vi "CleanDefaultInterfaces.vi"(8 "error in":errorcluster, 11 "Config in":T1) -> (0 "error out":errorcluster, 3 "Config out":T1)   [LabVIEW 2020]
uses:
  <vilib>/WebServerConfig/Config.ctl
  <vilib>/WebServerConfig/Server.ctl
  <vilib>/WebServerConfig/Alias.ctl
  <vilib>/WebServerConfig/ErrorDocument.ctl
  <vilib>/WebServerConfig/Action.ctl
  <vilib>/WebServerConfig/Redirect.ctl
  <vilib>/WebServerConfig/Interface.ctl
  <vilib>/WebServerConfig/AddHandler.ctl
  <vilib>/WebServerConfig/SSL.ctl
  <vilib>/WebServerConfig/CustomLog.ctl
  <vilib>/WebServerConfig/LoadModule.ctl
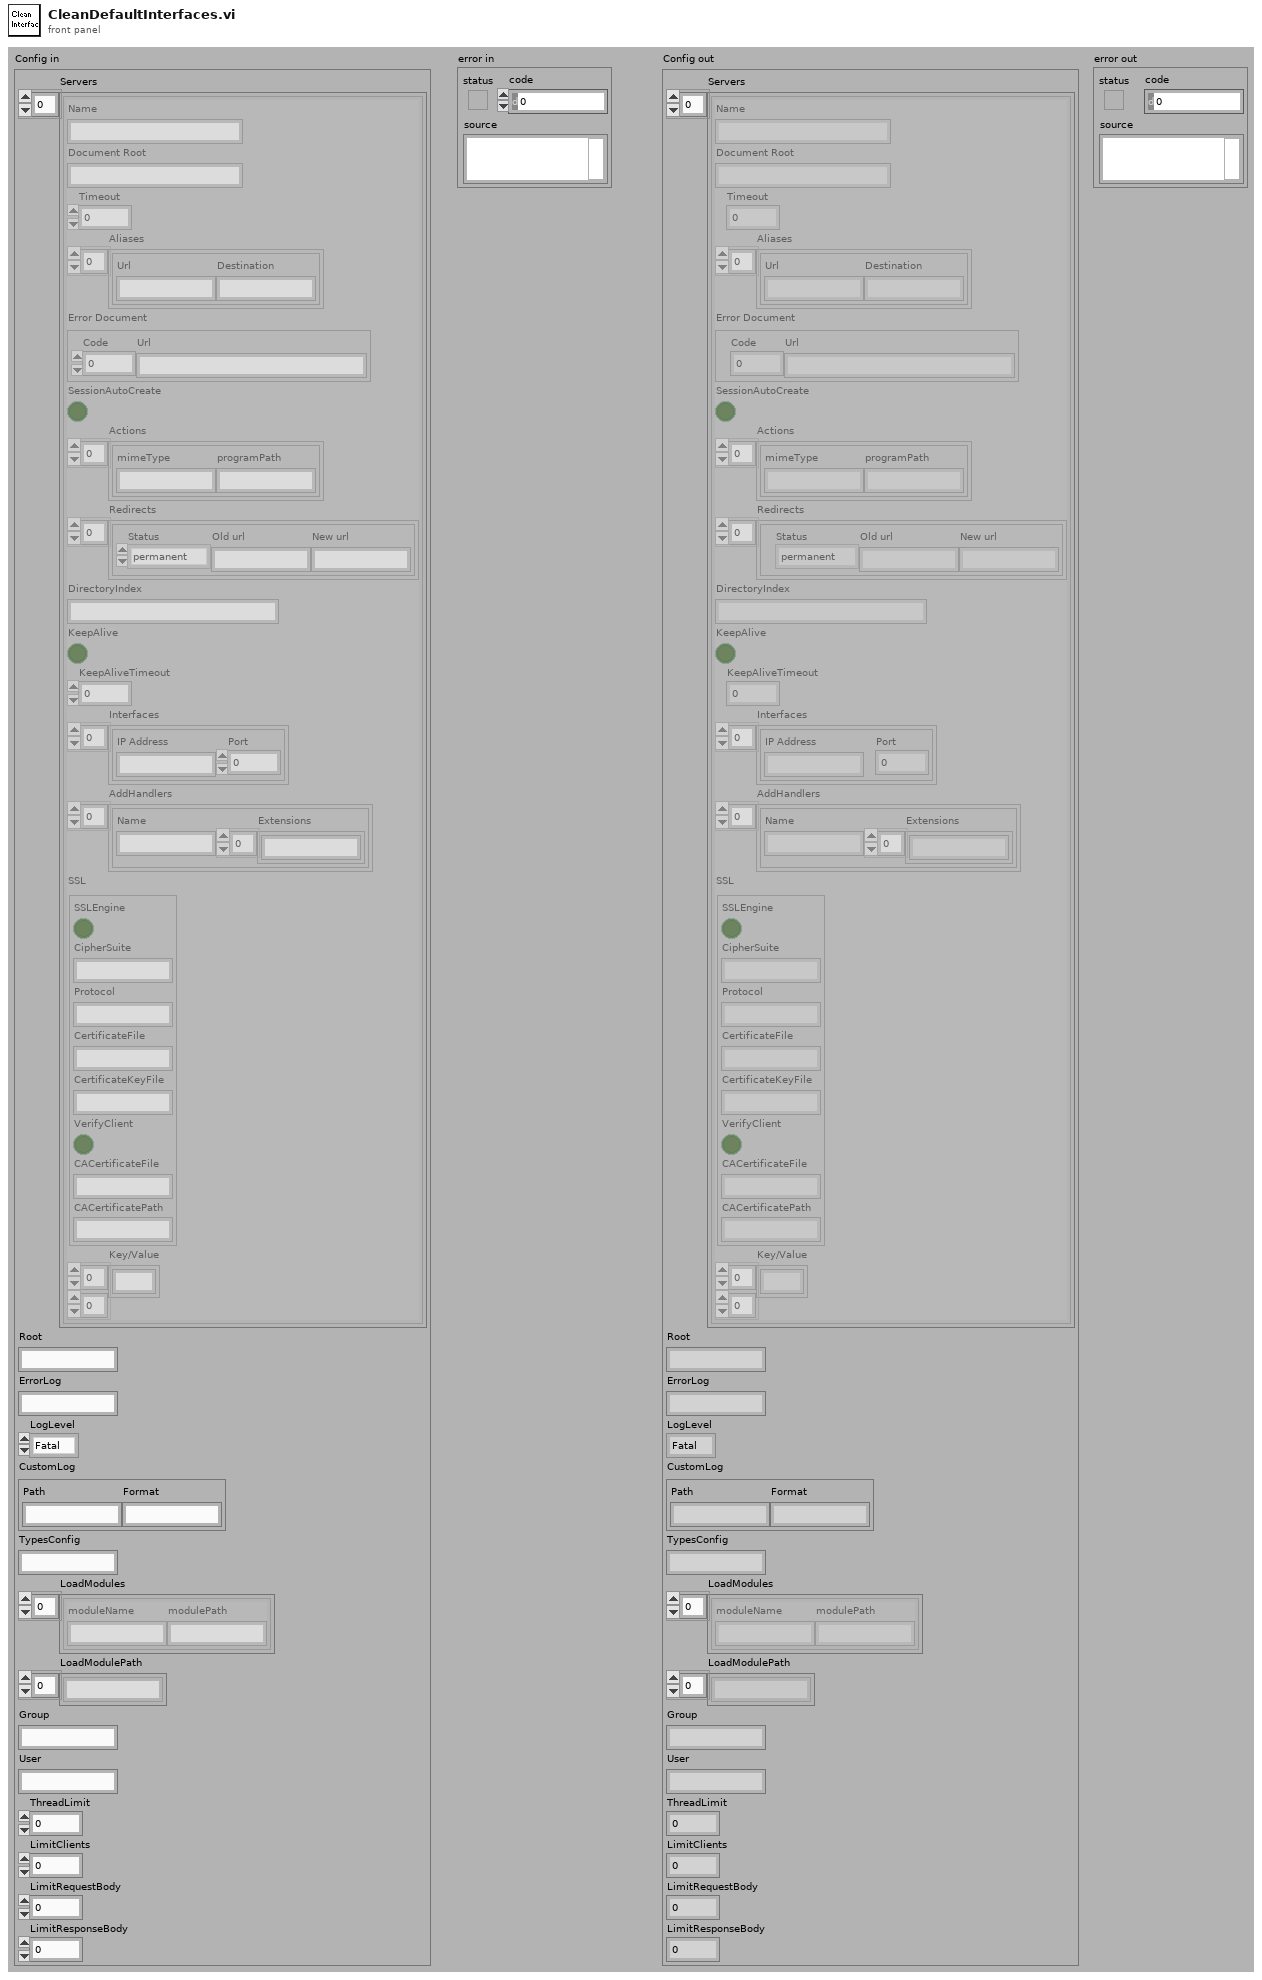
[diagram p1: front panel]
types:
  T1 = typedef "Config.ctl" = cluster{"Servers":T2[], "Root":string, "ErrorLog":string, "LogLevel":enum16{"Fatal", "Error", "Warn", "Info", "Debug", "5", "6", "7", "8", "Verbose"}, "CustomLog":T10, "TypesConfig":string, "LoadModules":T11[], "LoadModulePath":string[], "Group":string, "User":string, "ThreadLimit":u32, "LimitClients":u32, "LimitRequestBody":u32, "LimitResponseBody":u32}
  T2 = typedef "Server.ctl" = cluster{"Name":string, "Document Root":string, "Timeout":u32, "Aliases":T3[], "Error Document":T4, "SessionAutoCreate":bool, "Actions":T5[], "Redirects":T6[], "DirectoryIndex":string, "KeepAlive":bool, "KeepAliveTimeout":u32, "Interfaces":T7[], "AddHandlers":T8[], "SSL":T9, "Key/Value":string[][]}
  T3 = typedef "Alias.ctl" = cluster{"Url":string, "Destination":string}
  T4 = typedef "ErrorDocument.ctl" = cluster{"Code":u16, "Url":string}
  T5 = typedef "Action.ctl" = cluster{"mimeType":string, "programPath":string}
  T6 = typedef "Redirect.ctl" = cluster{"Status":enum16{"permanent", "temp", "seeother", "gone"}, "Old url":string, "New url":string}
  T7 = typedef "Interface.ctl" = cluster{"IP Address":string, "Port":u16}
  T8 = typedef "AddHandler.ctl" = cluster{"Name":string, "Extensions":string[]}
  T9 = typedef "SSL.ctl" = cluster{"SSLEngine":bool, "CipherSuite":string, "Protocol":string, "CertificateFile":string, "CertificateKeyFile":string, "VerifyClient":bool, "CACertificateFile":string, "CACertificatePath":string}
  T10 = typedef "CustomLog.ctl" = cluster{"Path":string, "Format":string}
  T11 = typedef "LoadModule.ctl" = cluster{"moduleName":string, "modulePath":string}
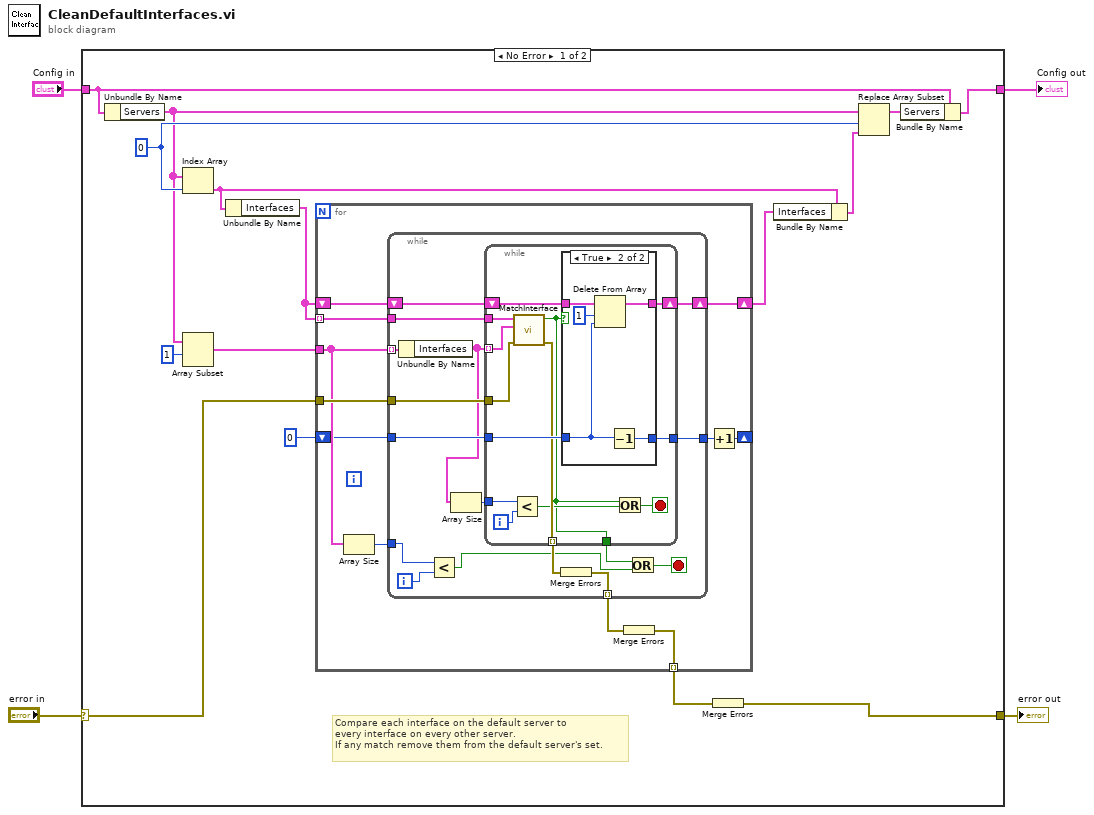
[diagram p0: block diagram]
diagram:
  n1 = case shown="No Error" "error in" {
    selector: "error in" -> [w6 w68]
    tunnel: [w19 w68] -> w4
    tunnel: [w11 w67] -> w3
    tunnel: "Config in" -> [w10 w67]
    frame No Error {
      w17 = 0 ("index")
      # "Compare each interface on the default server to\nevery interface on every other server.\nIf any match remove them from the default server's set."
      n2 = Unbundle By Name(w10) -> ("Servers"=w14:T2[])
      n3 = Index Array(array=w14, index=w17) -> (element=w13:T2)
      n4 = Array Subset(array=w14, index=1) -> (w8:T2[])  [unwired: 1 in]
      n5 = Unbundle By Name(w13) -> ("Interfaces"=w9:T7[])
      n6 = for {
        tunnel: w9 -> [w30] mode=indexing
        tunnel: w8 -> [w24]
        tunnel: w6 -> [w29]
        shift-right: [w27] -> w12
        shift-left: w9 -> [w28]
        tunnel: [w26] -> w18 mode=indexing
        shift-right: [w20] -> _
        shift-left: 0 -> [w22]
        n7 = Array Size(array=w24) -> (size(s)=w23:i32)
        n8 = while {
          tunnel: w24 -> [w46] mode=indexing
          tunnel: w30 -> [w45]
          tunnel: w29 -> [w44]
          tunnel: w22 -> [w43]
          tunnel: [w39] -> w25 mode=indexing
          shift-right: [w41] -> w27
          shift-left: w28 -> [w42]
          tunnel: w23 -> [w37]
          tunnel: [w31] -> w21
          i -> [w38]
          stop <- w36 stop-if-true
          n9 = Unbundle By Name(w46) -> ("Interfaces"=w34:T7[])
          n10 = Less?(x=w37, y=w38) -> (x < y?=w35:bool)
          n11 = Array Size(array=w34) -> (size(s)=w33:i32)
          n12 = while {
            tunnel: w34 -> [w58] mode=indexing
            tunnel: w45 -> [w59]
            tunnel: w44 -> [w57]
            tunnel: w43 -> [w56]
            tunnel: [w53] -> w40 mode=indexing
            shift-right: [w54] -> w41
            shift-left: w42 -> [w55]
            tunnel: w33 -> [w52]
            tunnel: [w48] -> w32
            tunnel: [w47] -> w31
            i -> [w51]
            stop <- w50 stop-if-true
            n13 = Less?(x=w52, y=w51) -> (x < y?=w49:bool)
            n14 = call <vilib>:"MatchInterface.vi"("error in (no error)"=w57, "Interface 2"=w58, "Interface 1"=w59) -> ("error out"=w53:errorcluster, "Matches"=w48:bool)  [unwired: 6 in, 1 out]
            n15 = case shown="True" w48 {
              tunnel: w56 -> [w60 w63]
              tunnel: w55 -> [w61 w66]
              tunnel: [w61 w64] -> w54
              tunnel: [w60 w62] -> w47
              frame False {
              }
              frame True {
                n16 = Delete From Array(array=w66, length=1, index=w63) -> (array with subset deleted=w64:T7[])  [unwired: 1 out]
                n17 = Decrement(x=w63) -> (x-1=w62:i32)
              }
            }
            n18 = Or(x=w48, y=w49) -> (x .or. y?=w50:bool)
          }
          n19 = Merge Errors(w40) -> (w39:errorcluster)
          n20 = Or(x=w32, y=w35) -> (x .or. y?=w36:bool)
        }
        n21 = Merge Errors(w25) -> (w26:errorcluster)
        n22 = Increment(x=w21) -> (x+1=w20:i32)
      }
      n23 = Merge Errors(w18) -> (w19:errorcluster)
      n24 = Bundle By Name(cluster=w13, "Interfaces"=w12) -> (w16:T2)
      n25 = Replace Array Subset(array=w14, new element=w16, index=w17) -> (w15:T2[])
      n26 = Bundle By Name(cluster=w10, "Servers"=w15) -> (w11:T1)
    }
    frame Error {
    }
  }
  "error out" <- w4
  "Config out" <- w3
